vi "Handle Error.vi"(8 "error in (no error)":errorcluster caption="错误输入（无错误）", 11 "HL7 in":refnum<class "HL7.lvclass"> caption="操作者输入") -> (0 "error out":errorcluster caption="错误输出", 2 "stop actor?":bool=TRUE caption="停止操作者？", 3 "HL7 out":refnum<class "HL7.lvclass"> caption="操作者输出")   [LabVIEW 2016, in "HL7.lvlib" / "HL7.lvclass"]
doc: "(<B>Filename</B>: Actor Framework.lvlib:Actor.lvclass:Handle Error.vi)\n\nDefines how the actor handles an error that occurred while processing a message.默认情况下，该方法不执行任何操作，仅停止操作者。"
uses:
  HL7.lvclass
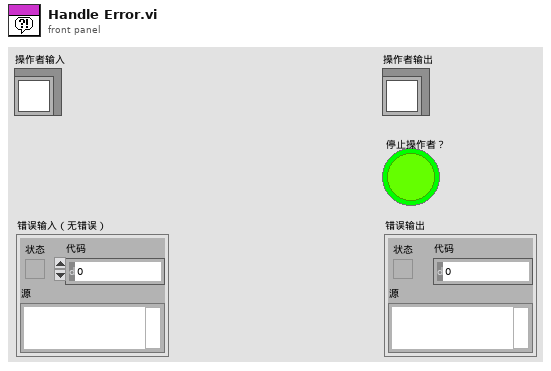
[diagram p1: front panel]
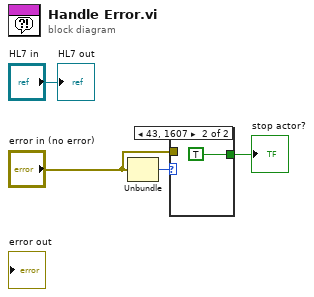
[diagram p0: block diagram]
diagram:
  n1 = Unbundle("error in (no error)") -> ("code"=w4:i32)  [unwired: 2 out]
  n2 = case shown="43, 1607" w4 {
    tunnel: "error in (no error)" -> [_ _]
    tunnel: [_ TRUE] -> w1
    frame Default {
    }
    frame 43, 1607 {
    }
  }
  "stop actor?" <- w1
  "HL7 out" <- "HL7 in"
